vi "Word to double.vi"(5 "ScaleOffset (0)":dbl, 7 "ScaleFac (1)":dbl=1.0, 8 "Word":bool[](array[boolean]), 9 "Signed? (F)":bool, 10 "Number of Bits":T2=1 min=1 max=32, 11 "Start Bit":T1) -> (3 "Double":dbl)   [LabVIEW 2017, in "Ballard Arinc-429 Shared.lvlib"]
uses:
  Ballard Arinc-429 Shared.lvlib
  Controls and Global/Number of Bits.ctl
  Controls and Global/Start Bit.ctl
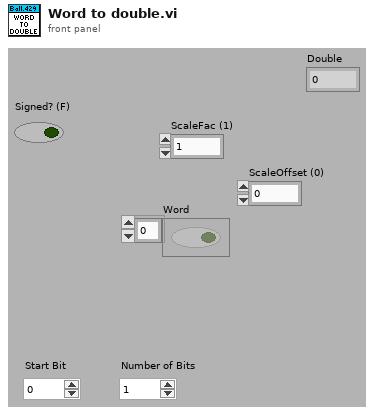
[diagram p1: front panel]
types:
  T1 = typedef "Ballard Arinc-429 Shared.lvlib/Start Bit.ctl" = i32
  T2 = typedef "Ballard Arinc-429 Shared.lvlib/Number of Bits.ctl" = i32
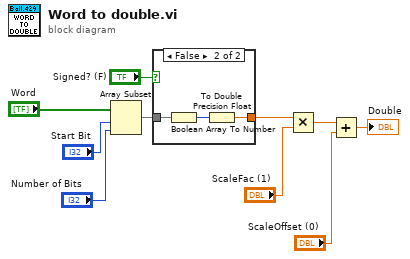
[diagram p0: block diagram]
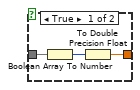
[diagram p2: hidden frame]
diagram:
  n1 = Array Subset(array="Word", index="Start Bit", length="Number of Bits") -> (w8:bool[])
  n2 = case shown="False" "Signed? (F)" {
    tunnel: w8 -> [w13 w16]
    tunnel: [w11 w14] -> w6
    frame True {
      n3 = Boolean Array To Number(Boolean array=w13) -> (number=w12:i32)
      n4 = To Double Precision Float(number=w12) -> (double precision float=w11:dbl)
    }
    frame False {
      n5 = Boolean Array To Number(Boolean array=w16) -> (number=w15:u32)
      n6 = To Double Precision Float(number=w15) -> (double precision float=w14:dbl)
    }
  }
  n7 = Multiply(x=w6, y="ScaleFac (1)") -> (x*y=w4:dbl)
  n8 = Add(x=w4, y="ScaleOffset (0)") -> (x+y=→"Double":dbl)
